vi "Get-sequence-step.vi"(8 "error in (no error)":errorcluster, 10 "Motor index":i32, 11 "Object ref in":T1) -> (0 "error out":errorcluster, 2 "Sequence step":i32, 3 "Object ref out":T1)   [LabVIEW 2013, in "PowderDeposition.lvlib" / "PD-Main.lvclass"]
uses:
  PD-Main.lvclass
  Object-reference.ctl
  PD-Main.lvclass/PD-Main.ctl
  Read Motor sequences.vi
  Write Sequence index.vi
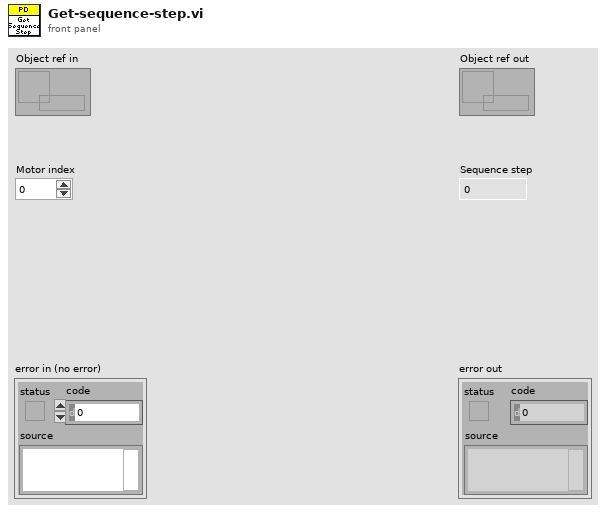
[diagram p1: front panel]
types:
  T1 = typedef "PowderDeposition.lvlib/PD-Main.lvclass/Object-reference.ctl" = refnum<data-value>
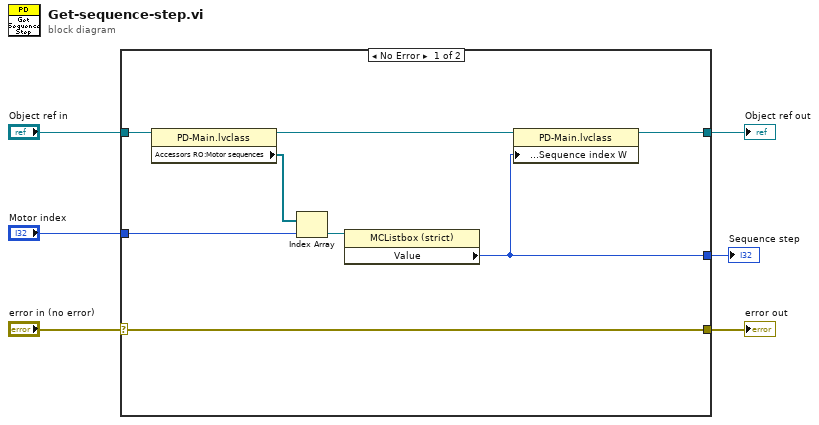
[diagram p0: block diagram]
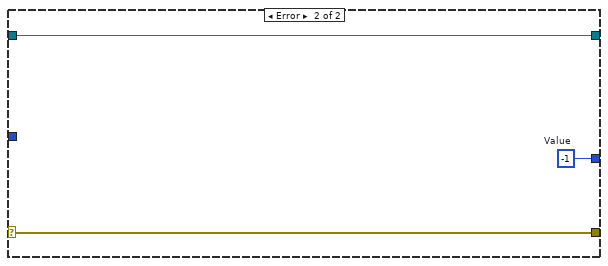
[diagram p2: hidden frame]
diagram:
  n1 = case shown="No Error" "error in (no error)" {
    selector: "error in (no error)" -> [w14 w17]
    tunnel: [w14 w17] -> w5
    tunnel: [w8 w16] -> w3
    tunnel: "Object ref in" -> [w13 w16]
    tunnel: "Motor index" -> [w10 _]
    tunnel: [w7 w15] -> w1
    frame No Error {
      n2 = property class="PD-Main.lvclass"(reference=w13) -> (reference out=w12:T1, "Accessors RO:Motor sequences"=w11:refnum<vi>[])  [unwired: 1 in, 1 out]
      n3 = Index Array(array=w11, index=w10) -> (element=w9:refnum<vi>)
      n4 = property class="MCListbox (strict)"(reference=w9) -> ("Value"=w7:i32)  [unwired: 1 in, 2 out]
      n5 = property class="PD-Main.lvclass"(reference=w12, "Accessors/Modifiers:Sequence index W"=w7) -> (reference out=w8:T1)  [unwired: 1 in, 1 out]
    }
    frame Error {
      w15 = -1  # Value
    }
  }
  "error out" <- w5
  "Object ref out" <- w3
  "Sequence step" <- w1
